vi "DestroyCommunication.vi"(8 "error in (no error)":errorcluster, 11 "Message Queues out":T1) -> (0 "error out":errorcluster)   [LabVIEW 2017, in "Server.lvlib" / "Message Queue.lvlib"]
doc: "Destroys all Queues and User Events."
uses:
  Message Queue.lvlib
  CommReferences.ctl
  MessageCluster.ctl
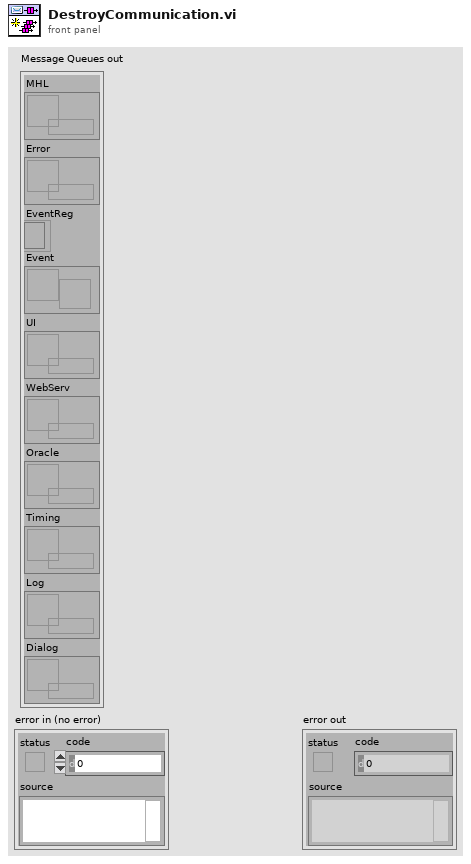
[diagram p1: front panel]
types:
  T1 = typedef "Server.lvlib/Message Queue.lvlib/CommReferences.ctl" = cluster{"MHL":refnum<queue>, "Error":refnum<queue>, "EventReg":refnum<event-registration>, "Event":refnum<user-event>, "UI":refnum<queue>, "WebServ":refnum<queue>, "Oracle":refnum<queue>, "Timing":refnum<queue>, "Log":refnum<queue>, "Dialog":refnum<queue>}
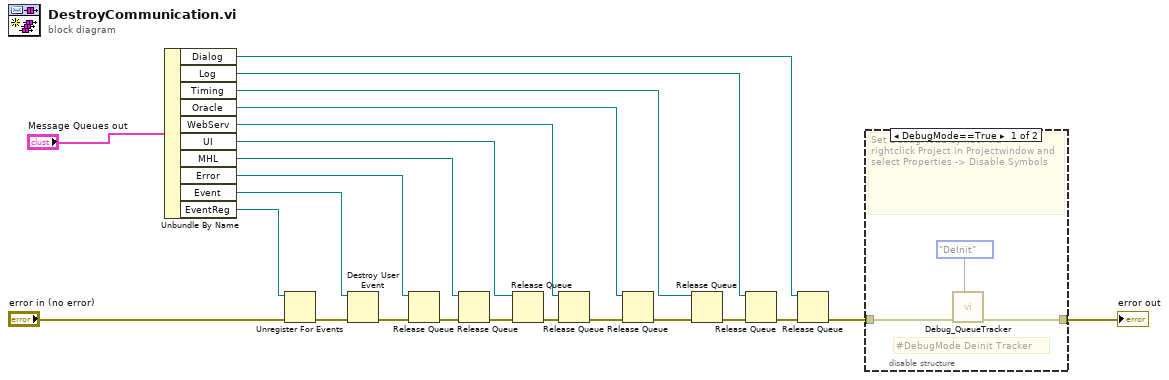
[diagram p0: block diagram]
diagram:
  n1 = Unbundle By Name("Message Queues out") -> ("Dialog"=w1:refnum<queue>, "Log"=w9:refnum<queue>, "Timing"=w10:refnum<queue>, "Oracle"=w11:refnum<queue>, "WebServ"=w12:refnum<queue>, "UI"=w13:refnum<queue>, "MHL"=w15:refnum<queue>, "Error"=w16:refnum<queue>, "Event"=w18:refnum<user-event>, "EventReg"=w20:refnum<event-registration>)
  n2 = Unregister For Events(event registration refnum=w20, error in="error in (no error)") -> (error out=w21:errorcluster)
  n3 = Destroy User Event(user event=w18, error in=w21) -> (error out=w19:errorcluster)
  n4 = Release Queue(queue=w16, error in (no error)=w19) -> (error out=w17:errorcluster)  [unwired: 1 in, 2 out]
  n5 = Release Queue(queue=w15, error in (no error)=w17) -> (error out=w8:errorcluster)  [unwired: 1 in, 2 out]
  n6 = Release Queue(queue=w13, error in (no error)=w8) -> (error out=w7:errorcluster)  [unwired: 1 in, 2 out]
  n7 = Release Queue(queue=w12, error in (no error)=w7) -> (error out=w6:errorcluster)  [unwired: 1 in, 2 out]
  n8 = Release Queue(queue=w11, error in (no error)=w6) -> (error out=w5:errorcluster)  [unwired: 1 in, 2 out]
  n9 = Release Queue(queue=w10, error in (no error)=w5) -> (error out=w4:errorcluster)  [unwired: 1 in, 2 out]
  n10 = Release Queue(queue=w9, error in (no error)=w4) -> (error out=w3:errorcluster)  [unwired: 1 in, 2 out]
  n11 = Release Queue(queue=w1, error in (no error)=w3) -> (error out=w2:errorcluster)  [unwired: 1 in, 2 out]
  n12 = disable-structure shown="DebugMode==True" {
    disable-tunnel: [w26 w27] -> w14
    disable-tunnel: w2 -> [w24 w27]
    frame condition #0 {
      # "#DebugMode Deinit Tracker"
      # "Set DebugMode-Symbol via\nrightclick Project in Projectwindow and select Properties -> Disable Symbols"
      n13 = call "Debug_QueueTracker.vi"("Mode"=enum16{"Init", "Track", "DeInit"}."DeInit", "Error In"=w24) -> ("Error Out"=w26:errorcluster)  [unwired: 9 in]
    }
    frame condition #1 (active) {
      # "Don't track Queues if not in \nDebug-Mode.\nMode is settable in Project-file"
    }
  }
  "error out" <- w14
